vi "prepAO_sealtest.vi"   [LabVIEW 2013]
uses:
  <vilib>/DAQmx/write.llb/DAQmx Write (Analog 1D DBL 1Chan NSamp).vi
  <vilib>/DAQmx/write.llb/DAQmx Write (Analog 2D DBL NChan NSamp).vi
  <vilib>/DAQmx/create/channels.llb/DAQmx Create Channel (AO-Voltage-Basic).vi
  <vilib>/DAQmx/configure/timing.llb/DAQmx Timing (Sample Clock).vi
  <vilib>/DAQmx/miscellaneous.llb/DAQmx Fill In Error Info.vi
  <resource>/objmgr/daqmx.rc
types:
  T1 = cluster{"Min Voltage sq (mV)":dbl, "Max voltage sq (mV)":dbl, "Duty cycle sq(%)":dbl, "Voltage freq. sq(Hz)":dbl, "# cycles sq":u32, "meastype":enum16{"sealtest hekcells", "sealtest neurons", "Manual", "from file"}, "sample rate":dbl, "amp":dbl, "sample mode":i32, "refreshbuffer":i32, "timeout":sgl, "patch":bool, "laserAO":bool, "shutter":bool, "488":bool, "532":bool, "640":bool, "Vhold":dbl, "holdon":bool, "Min Voltage tri (mV)":dbl, "Max voltage tri (mV)":dbl, "Voltage freq. tri(Hz)":dbl, "# cycles tri":u32, "Voltage step ":bool, "Voltage triangle":bool, "file":bool}
  T2 = cluster{"CH1 AI":tag, "CH1 CI":tag, "CH2 AI":tag, "CH2 CI":tag, "AI X":tag, "AI Y":tag, "AO X-Y":tag, "CH1ST":bool, "CH2ST":bool, "Sigcase":i16, "StageS":i32, "StageL":i32, "data dir":path, "AI VC":tag, "AI CC":tag, "AO CWlaser":tag, "AO VtoP":tag, "shutter":tag, "488":tag, "532":tag, "640":tag}
  T3 = cluster{"Xpixels":i32, "Vx-min ref":dbl, "Vx-max ref":dbl, "Ypixels":i32, "Vy-min ref":dbl, "Vy-max ref":dbl, "srate":dbl, "type":string, "date":string, "time":string, "Colormap":u16, "square pixels":bool, "square matrix":bool, "Xpixels Img":i32, "Vx-min Img":dbl, "VX-max Img":dbl, "Ypixels Img":i32, "Vy-min Img":dbl, "Vy-max Img ":dbl, "autoshutter":bool, "P":dbl, "sAOxy":i32, "finite":bool, "cont":bool, "wavdet":bool, "measpoints":i32, "avpp":i32, "bufferAO":i32, "bufferAI":i32, "CH1":bool, "CH2":bool, "X":bool, "Y":bool, "timeout":dbl, "starttick":u32, "waveform":path, "Vy-ref":dbl, "Vx-ref":dbl, "refreshrate":dbl, "refreshbuffer":i32, "tt_cycles":i32, "motorref":refnum<k7>, "mirrorswitch":refnum<k7>, "sample mode":i32}
  T4 = cluster{"VtoP":dbl[], "CWlasers":dbl[], "shutter":dbl[], "488":dbl[], "532":dbl[], "640":dbl[]}
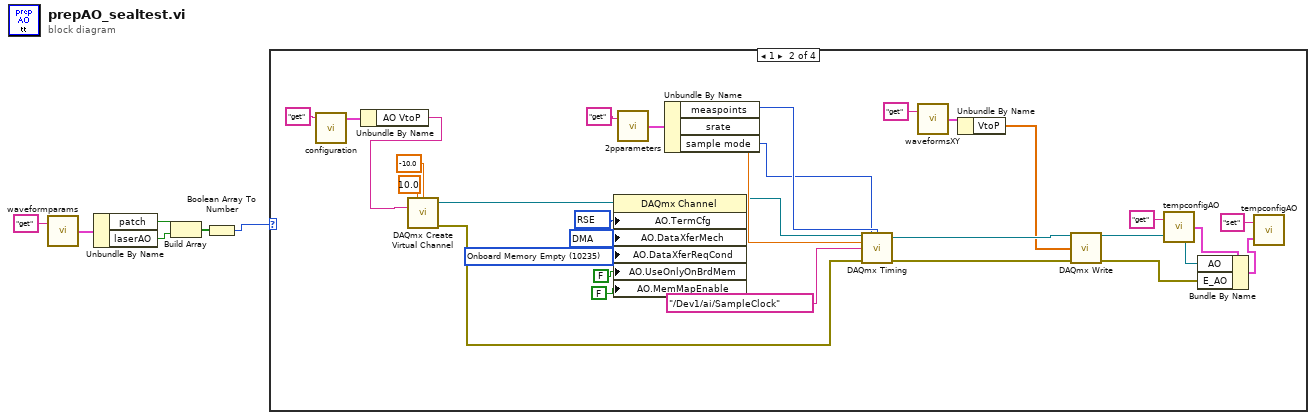
[diagram p0: block diagram]
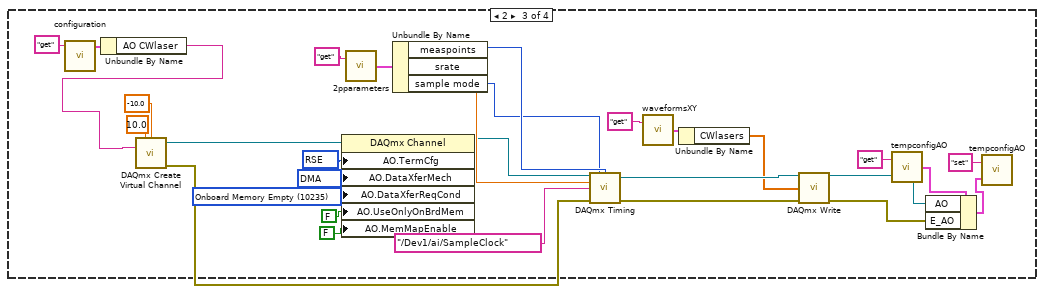
[diagram p3: hidden frame]
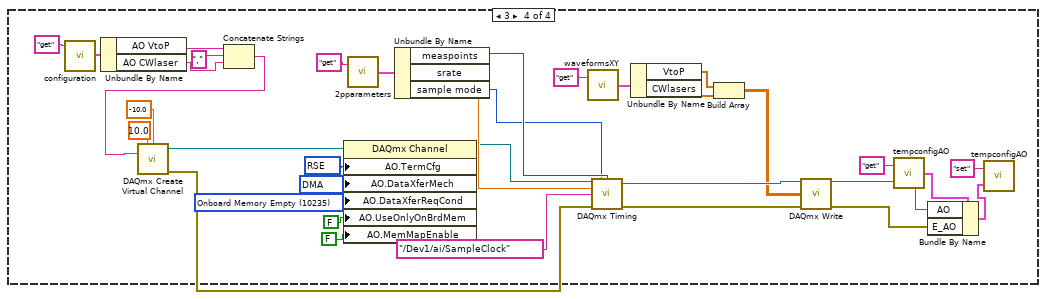
[diagram p4: hidden frame]
diagram:
  n1 = call "waveformparams.vi"("command"="get") -> ("Params out"=w4:T1)  [unwired: 1 in]
  n2 = Unbundle By Name(w4) -> ("patch"=w3:bool, "laserAO"=w2:bool)
  n3 = Build Array(w3, w2) -> (w1:bool[])
  n4 = Boolean Array To Number(Boolean array=w1) -> (number=w6:u32)
  n5 = case shown="1" w6 {
    frame 0, Default {
    }
    frame 1 {
      w17 = 10235 items=["Onboard Memory Empty"=10235, "Onboard Memory Half Full or Less"=10239, "Onboard Memory Less than Full"=10242] ("AO.DataXferReqCond 2")
      w16 = 10054 items=["DMA"=10054, "Interrupts"=10204, "Programmed I/O"=10264, "USB Bulk"=12590] ("AO.DataXferMech 2")
      w15 = 10083 items=["RSE"=10083, "Differential"=10106, "Pseudodifferential"=12529] ("AO.TermCfg")
      n6 = call "configuration.vi"("command"="get") -> ("config out"=w9:T2)  [unwired: 2 in, 1 out]
      n7 = Unbundle By Name(w9) -> ("AO VtoP"=w7:tag)
      n8 = call-poly <vilib>:"DAQmx Create Virtual Channel.vi"("maximum value"=10.0, "minimum value"=-10.0, "physical channels"=w7) -> ("task out"=w22:refnum<k21>, "error out"=w32:errorcluster)  [unwired: 6 in, 5 out]
      n9 = property class="DAQmx Channel"(reference=w22, "AO.TermCfg"=w15, "AO.DataXferMech"=w16, "AO.DataXferReqCond"=w17, "AO.UseOnlyOnBrdMem"=FALSE, "AO.MemMapEnable"=FALSE) -> (reference out=w23:refnum<k21>)  [unwired: 1 in, 1 out]
      n10 = call "2pparameters.vi"("command"="get") -> ("Params out"=w25:T3)  [unwired: 1 in]
      n11 = Unbundle By Name(w25) -> ("measpoints"=w27:i32, "srate"=w36:dbl, "sample mode"=w13:i32)
      n12 = call-poly <vilib>:"DAQmx Timing.vi"("task/channels in"=w23, "sample mode"=w13, "samples per channel"=w27, "rate"=w36, "source"=tag "/Dev1/ai/SampleClock", "error in"=w32) -> ("task out"=w24:refnum<k21>, "error out"=w33:errorcluster)  [unwired: 1 in, 7 out]
      n13 = call "waveformsXY.vi"("command"="get") -> ("waveforms out"=w12:T4)  [unwired: 1 in]
      n14 = Unbundle By Name(w12) -> ("VtoP"=w10:dbl[])
      n15 = call-poly <vilib>:"DAQmx Write.vi"("task/channels in"=w24, "data"=w10, "error in"=w33) -> ("task out"=w35:refnum<k21>, "error out"=w34:errorcluster)  [unwired: 10 in, 1 out]
      n16 = call "tempconfigAO.vi"("command"="get") -> ("Temp Config out"=w30:cluster{"AO":refnum<k21>, "E_AO":errorcluster})  [unwired: 1 in]
      n17 = Bundle By Name(cluster=w30, "AO"=w35, "E_AO"=w34) -> (w31:cluster{"AO":refnum<k21>, "E_AO":errorcluster})
      n18 = call "tempconfigAO.vi"("Temp Config in"=w31, "command"="set") -> ()  [unwired: 1 out]
    }
    frame 2 {
      w47 = 10235 items=["Onboard Memory Empty"=10235, "Onboard Memory Half Full or Less"=10239, "Onboard Memory Less than Full"=10242] ("AO.DataXferReqCond 2")
      w46 = 10054 items=["DMA"=10054, "Interrupts"=10204, "Programmed I/O"=10264, "USB Bulk"=12590] ("AO.DataXferMech 2")
      w45 = 10083 items=["RSE"=10083, "Differential"=10106, "Pseudodifferential"=12529] ("AO.TermCfg")
      n19 = call "configuration.vi"("command"="get") -> ("config out"=w39:T2)  [unwired: 2 in, 1 out]
      n20 = Unbundle By Name(w39) -> ("AO CWlaser"=w37:tag)
      n21 = call-poly <vilib>:"DAQmx Create Virtual Channel.vi"("maximum value"=10.0, "minimum value"=-10.0, "physical channels"=w37) -> ("task out"=w52:refnum<k21>, "error out"=w62:errorcluster)  [unwired: 6 in, 5 out]
      n22 = property class="DAQmx Channel"(reference=w52, "AO.TermCfg"=w45, "AO.DataXferMech"=w46, "AO.DataXferReqCond"=w47, "AO.UseOnlyOnBrdMem"=FALSE, "AO.MemMapEnable"=FALSE) -> (reference out=w53:refnum<k21>)  [unwired: 1 in, 1 out]
      n23 = call "2pparameters.vi"("command"="get") -> ("Params out"=w55:T3)  [unwired: 1 in]
      n24 = Unbundle By Name(w55) -> ("measpoints"=w57:i32, "srate"=w66:dbl, "sample mode"=w43:i32)
      n25 = call-poly <vilib>:"DAQmx Timing.vi"("task/channels in"=w53, "sample mode"=w43, "samples per channel"=w57, "rate"=w66, "source"=tag "/Dev1/ai/SampleClock", "error in"=w62) -> ("task out"=w54:refnum<k21>, "error out"=w63:errorcluster)  [unwired: 1 in, 7 out]
      n26 = call "waveformsXY.vi"("command"="get") -> ("waveforms out"=w42:T4)  [unwired: 1 in]
      n27 = Unbundle By Name(w42) -> ("CWlasers"=w40:dbl[])
      n28 = call-poly <vilib>:"DAQmx Write.vi"("task/channels in"=w54, "data"=w40, "error in"=w63) -> ("task out"=w65:refnum<k21>, "error out"=w64:errorcluster)  [unwired: 10 in, 1 out]
      n29 = call "tempconfigAO.vi"("command"="get") -> ("Temp Config out"=w60:cluster{"AO":refnum<k21>, "E_AO":errorcluster})  [unwired: 1 in]
      n30 = Bundle By Name(cluster=w60, "AO"=w65, "E_AO"=w64) -> (w61:cluster{"AO":refnum<k21>, "E_AO":errorcluster})
      n31 = call "tempconfigAO.vi"("Temp Config in"=w61, "command"="set") -> ()  [unwired: 1 out]
    }
    frame 3 {
      w82 = 10235 items=["Onboard Memory Empty"=10235, "Onboard Memory Half Full or Less"=10239, "Onboard Memory Less than Full"=10242] ("AO.DataXferReqCond 2")
      w81 = 10054 items=["DMA"=10054, "Interrupts"=10204, "Programmed I/O"=10264, "USB Bulk"=12590] ("AO.DataXferMech 2")
      w80 = 10083 items=["RSE"=10083, "Differential"=10106, "Pseudodifferential"=12529] ("AO.TermCfg")
      n32 = call "configuration.vi"("command"="get") -> ("config out"=w71:T2)  [unwired: 2 in, 1 out]
      n33 = Unbundle By Name(w71) -> ("AO VtoP"=w69:tag, "AO CWlaser"=w68:tag)
      n34 = Concatenate Strings(w69, "," ("string"), w68) -> (w67:string)
      n35 = call-poly <vilib>:"DAQmx Create Virtual Channel.vi"("maximum value"=10.0, "minimum value"=-10.0, "physical channels"=w67) -> ("task out"=w87:refnum<k21>, "error out"=w97:errorcluster)  [unwired: 6 in, 5 out]
      n36 = property class="DAQmx Channel"(reference=w87, "AO.TermCfg"=w80, "AO.DataXferMech"=w81, "AO.DataXferReqCond"=w82, "AO.UseOnlyOnBrdMem"=FALSE, "AO.MemMapEnable"=FALSE) -> (reference out=w88:refnum<k21>)  [unwired: 1 in, 1 out]
      n37 = call "2pparameters.vi"("command"="get") -> ("Params out"=w90:T3)  [unwired: 1 in]
      n38 = Unbundle By Name(w90) -> ("measpoints"=w92:i32, "srate"=w101:dbl, "sample mode"=w78:i32)
      n39 = call "waveformsXY.vi"("command"="get") -> ("waveforms out"=w74:T4)  [unwired: 1 in]
      n40 = call-poly <vilib>:"DAQmx Timing.vi"("task/channels in"=w88, "sample mode"=w78, "samples per channel"=w92, "rate"=w101, "source"=tag "/Dev1/ai/SampleClock", "error in"=w97) -> ("task out"=w89:refnum<k21>, "error out"=w98:errorcluster)  [unwired: 1 in, 7 out]
      n41 = Unbundle By Name(w74) -> ("VtoP"=w75:dbl[], "CWlasers"=w76:dbl[])
      n42 = Build Array(w75, w76) -> (w77:dbl[][])
      n43 = call-poly <vilib>:"DAQmx Write.vi"("task/channels in"=w89, "data"=w77, "error in"=w98) -> ("task out"=w100:refnum<k21>, "error out"=w99:errorcluster)  [unwired: 10 in, 1 out]
      n44 = call "tempconfigAO.vi"("command"="get") -> ("Temp Config out"=w95:cluster{"AO":refnum<k21>, "E_AO":errorcluster})  [unwired: 1 in]
      n45 = Bundle By Name(cluster=w95, "AO"=w100, "E_AO"=w99) -> (w96:cluster{"AO":refnum<k21>, "E_AO":errorcluster})
      n46 = call "tempconfigAO.vi"("Temp Config in"=w96, "command"="set") -> ()  [unwired: 1 out]
    }
  }
